vi "Set Path Name.vi"(8 "error in (no error)":errorcluster, 10 "Path":path, 11 "Report.lvclass in":refnum<class "Wind Report.lvclass">) -> (0 "error out":errorcluster, 3 "Report.lvclass out":refnum<class "Wind Report.lvclass">)   [LabVIEW 2009, in "Wind Report.lvclass"]
doc: "This parent method sets object data and can operate on the child object.\n\nAAL 9/09"
uses:
  Wind Report.lvclass
  Wind Report.lvclass/Wind Report.ctl
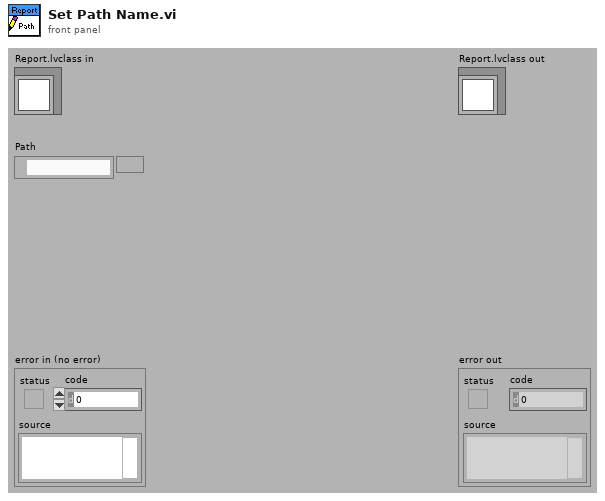
[diagram p1: front panel]
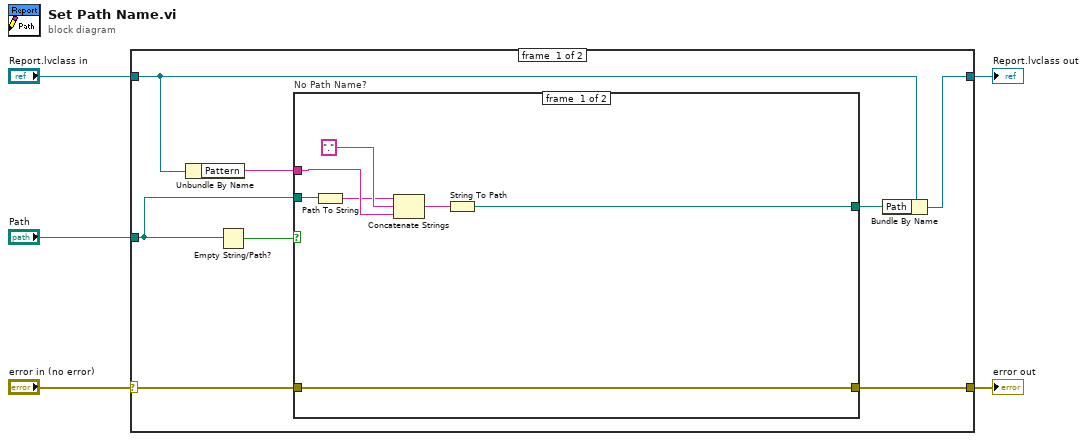
[diagram p0: block diagram]
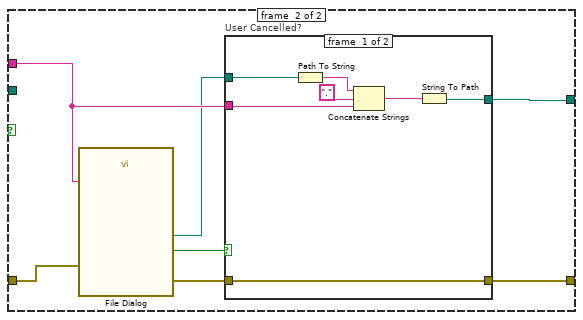
[diagram p2: hidden frame]
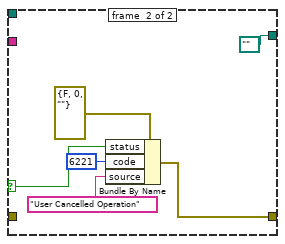
[diagram p3: hidden frame]
diagram:
  n1 = case shown="No Error" "error in (no error)" {
    selector: "error in (no error)" -> [w7 w41]
    tunnel: [w6 w41] -> w4
    tunnel: [w13 w42] -> w2
    tunnel: "Report.lvclass in" -> [w9 w42]
    tunnel: "Path" -> [w10 _]
    frame #0 {
      n2 = Unbundle By Name(w9) -> ("Pattern"=w8:string)
      n3 = Empty String/Path?(string/path=w10) -> (empty?=w12:bool)
      n4 = case "No Path Name?" shown="False" w12 {
        tunnel: [w16 w25] -> w11
        tunnel: w10 -> [w19 _]
        tunnel: w8 -> [w15 w24]
        tunnel: w7 -> [w20 w22]
        tunnel: [w20 w26] -> w6
        frame #0 {
          n5 = Path To String(path=w19) -> (string=w14:string)
          n6 = Concatenate Strings(w14, "." ("string"), w15) -> (w17:string)
          n7 = String To Path(string=w17) -> (path=w16:path)
        }
        frame #1 {
          n8 = call "File Dialog"("error in"=w22, "pattern (all files)"=w24) -> ("selected path"=w23:path, "cancelled"=w27:bool, "error out"=w21:errorcluster)  [unwired: 5 in, 6 out]
          n9 = case "User Cancelled?" shown="False" w27 {
            selector: w27 -> [_ w39]
            tunnel: [w34 w36] -> w26
            tunnel: w21 -> [w34 _]
            tunnel: [w28 path ""] -> w25
            tunnel: w24 -> [w30 _]
            tunnel: w23 -> [w29 _]
            frame #0 {
              n10 = Path To String(path=w29) -> (string=w32:string)
              n11 = Concatenate Strings(w32, "." ("string"), w30) -> (w31:string)
              n12 = String To Path(string=w31) -> (path=w28:path)
            }
            frame #1 {
              n13 = Bundle By Name(cluster=errorcluster {"status"=FALSE, "code"=0, "source"=""} ("error"), "status"=w39, "code"=6221, "source"="User Cancelled Operation") -> (w36:errorcluster)
            }
          }
        }
      }
      n14 = Bundle By Name(cluster=w9, "Path"=w11) -> (w13:refnum<class "Wind Report.lvclass">)
    }
    frame #1 {
    }
  }
  "error out" <- w4
  "Report.lvclass out" <- w2
